vi "Create VariantBuffer.vi"(5 "Buffer":refnum<class "VariantBuffer.lvclass">, 6 "buffer-type":T1, 7 "Allow Overflow?":bool=TRUE caption="Allow Overflow? (T)", 8 "error in":errorcluster, 10 "default":variant, 11 "bufSize":i32) -> (0 "error out":errorcluster, 3 "Buffer":refnum<data-value>)   [LabVIEW 2013, in "CircularBuffer.lvlib" / "VariantBuffer.lvclass"]
doc: "This VI creates a ring buffer of set size. This buffer is created in one place in the memory and is then accessed via pointer/reference.\n\nThe Data Type input is required because it defines the place in the memory to correct size thus removing the need for memory reallocation."
uses:
  VariantBuffer.lvclass
  buffer-type -- enum.ctl
  buffer-errors -- ring.ctl
  buffer-event -- enum.ctl
  VariantBuffer.lvclass/VariantBuffer.ctl
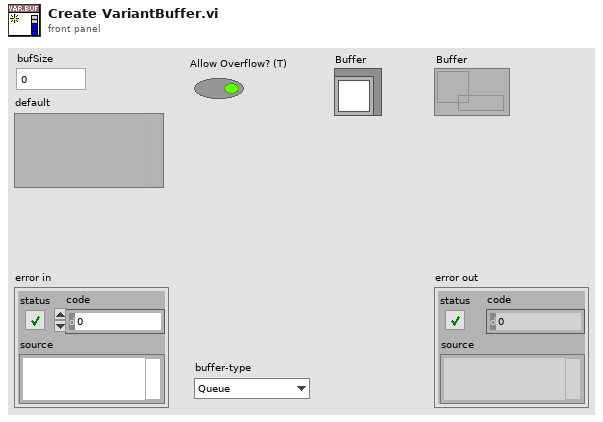
[diagram p1: front panel]
types:
  T1 = typedef "CircularBuffer.lvlib/VariantBuffer.lvclass/buffer-type -- enum.ctl" = enum16{"Queue", "Stack"}
  T2 = typedef "CircularBuffer.lvlib/VariantBuffer.lvclass/buffer-event -- enum.ctl" = enum16{"element-added", "element-removed", "filled", "emptied", "resized", "default-changed", "destroyed"}
  T3 = typedef "CircularBuffer.lvlib/VariantBuffer.lvclass/buffer-errors -- ring.ctl" = i32
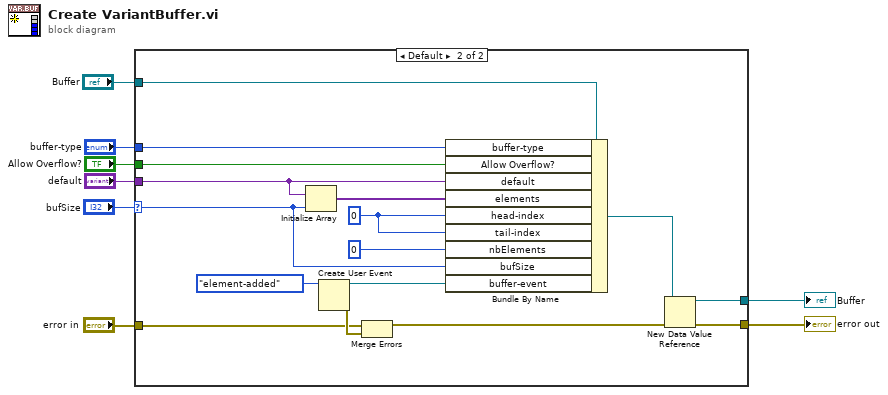
[diagram p0: block diagram]
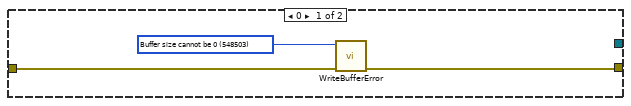
[diagram p2: hidden frame]
diagram:
  n1 = case shown="Default" "bufSize" {
    selector: "bufSize" -> [_ w12]
    tunnel: "Buffer" -> [_ w27]
    tunnel: [w9 w25] -> w7
    tunnel: [_ w24] -> w6
    tunnel: "default" -> [_ w23]
    tunnel: "Allow Overflow?" -> [_ w22]
    tunnel: "error in" -> [w11 w17]
    tunnel: "buffer-type" -> [_ w15]
    frame 0 {
      w10 = T3 548503 items=["No error"=0, "Generic Buffer error"=548500, "Buffer is full"=548501, "Buffer is empty"=548502, "Buffer size cannot be 0"=548503, "Buffer reference is invalid"=548504, "Buffer event reference invalid"=548505, "Buffer Type not supported"=548506, "Not enough space in the buffer for this operation"=548507] ("buffer-errors")
      n2 = call "WriteBufferError.vi"("error in (no error)"=w11, "buffer-errors"=w10) -> ("error out"=w9:errorcluster)  [unwired: 9 in]
    }
    frame Default {
      w14 = 0 ("Index")
      n3 = Initialize Array(w23, w12) -> (w26:variant[])
      n4 = Create User Event(user event datatype=buffer-event_--_enum."element-added" ("buffer-event")) -> (user event=w19:refnum<user-event>, error out=w18:errorcluster)  [unwired: 1 in]
      n5 = Merge Errors(w17, w18) -> (w16:errorcluster)
      n6 = Bundle By Name(cluster=w27, "buffer-type"=w15, "Allow Overflow?"=w22, "default"=w23, "elements"=w26, "head-index"=w14, "tail-index"=w14, "nbElements"=0, "bufSize"=w12, "buffer-event"=w19) -> (w20:refnum<class "VariantBuffer.lvclass">)
      n7 = New Data Value Reference(data value=w20, error in=w16) -> (data value reference=w24:refnum<data-value>, error out=w25:errorcluster)
    }
  }
  "error out" <- w7
  "Buffer" <- w6
